vi "PAQmem-RemoveZero.vi"(2 "OneTagData in":T1) -> (7 "OneTagData out":T1)   [LabVIEW 2020, in "PAQ-memory.lvclass"]
doc: "Remove entries with invalid zero time data"
uses:
  PAQ-memory.lvclass
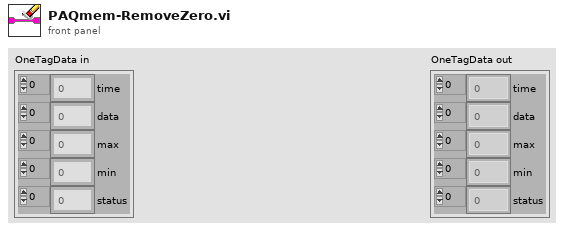
[diagram p1: front panel]
types:
  T1 = cluster{"time":dbl[], "data":dbl[], "max":dbl[], "min":dbl[], "status":u32[]}
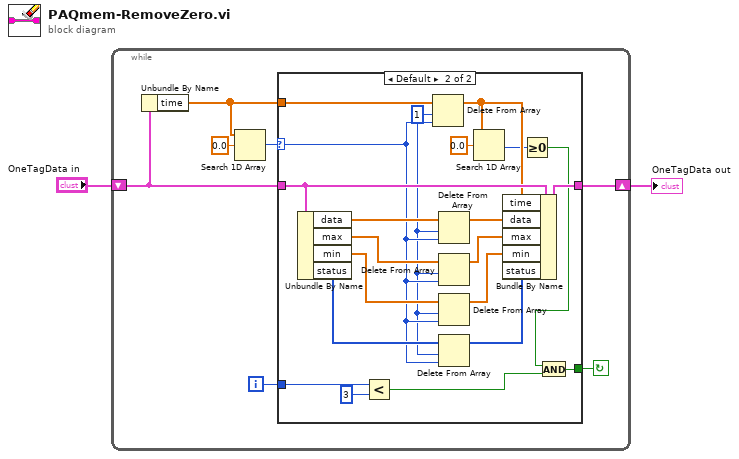
[diagram p0: block diagram]
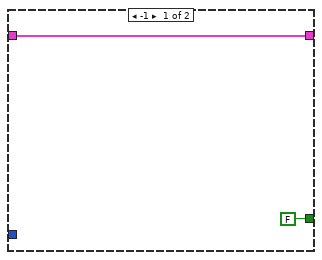
[diagram p2: hidden frame]
diagram:
  n1 = while {
    shift-right: [w5] -> w1
    shift-left: "OneTagData in" -> [w6]
    i -> [w3]
    stop <- w4 continue-if-true
    n2 = Unbundle By Name(w6) -> ("time"=w8:dbl[])
    n3 = Search 1D Array(1D array=w8, element=0.0) -> (index of element=w7:i32)  [unwired: 1 in]
    n4 = case shown="Default" w7 {
      selector: w7 -> [_ w21]
      tunnel: w8 -> [_ w32]
      tunnel: w6 -> [w11 w31]
      tunnel: [w11 w30] -> w5
      tunnel: [FALSE w17] -> w4
      tunnel: w3 -> [_ w19]
      frame -1 {
      }
      frame Default {
        w20 = 1 ("length")
        n5 = Unbundle By Name(w31) -> ("data"=w29:dbl[], "max"=w28:dbl[], "min"=w27:dbl[], "status"=w26:u32[])
        n6 = Less?(x=w19, y=3) -> (x < y?=w12:bool)
        n7 = Delete From Array(array=w32, length=w20, index=w21) -> (array with subset deleted=w15:dbl[])  [unwired: 1 out]
        n8 = Delete From Array(array=w29, length=w20, index=w21) -> (array with subset deleted=w25:dbl[])  [unwired: 1 out]
        n9 = Delete From Array(array=w28, length=w20, index=w21) -> (array with subset deleted=w24:dbl[])  [unwired: 1 out]
        n10 = Delete From Array(array=w27, length=w20, index=w21) -> (array with subset deleted=w23:dbl[])  [unwired: 1 out]
        n11 = Delete From Array(array=w26, length=w20, index=w21) -> (array with subset deleted=w22:u32[])  [unwired: 1 out]
        n12 = Search 1D Array(1D array=w15, element=0.0) -> (index of element=w14:i32)  [unwired: 1 in]
        n13 = Bundle By Name(cluster=w31, "time"=w15, "data"=w25, "max"=w24, "min"=w23, "status"=w22) -> (w30:T1)
        n14 = Greater Or Equal To 0?(x=w14) -> (x >= 0?=w13:bool)
        n15 = And(x=w13, y=w12) -> (x .and. y?=w17:bool)
      }
    }
  }
  "OneTagData out" <- w1
